vi "Get Physical Units from TD__ogtk.vi"(8 "error in (no error)":errorcluster, 10 "Float or Array Type Descriptor":T2) -> (0 "error out":errorcluster, 2 "Physical Units":T1[](array[typedef]))   [LabVIEW 2011]
doc: "Returns the physical units of the TD (number or array)."
uses:
  Type Descriptor__ogtk.ctl
  Physical Units__ogtk.ctl
panel:
  in  "Physical Units (type)":T1
  # "[OpenG VI Tags] ***Do Not Remove***"
  # "Please visit http://www.OpenG.org to learn about the\nOpen Source LabVIEW software movement.\n\nNOTICE -- YOU MUST LEAVE THIS NOTICE IN PLACE.  PER THE TERMS OF THE LICENSE BELOW, YOU MAY SUBLICENSE THIS SOFTWARE \nIN ANY WAY THAT DOES NOT CONFLICT WITH THIS LICENSE.\n\n### BSD License (http://www.opensource.org/licenses/bsd-license.php) Begin ###\n \nCopyright (c) 2002, Jean-Pierre Drolet <drolet_jp@hotmail.com>\nCopyright (c) 2002-2006, Jim Kring <jim@jimkring.com>\n\nAll rights reserved.\n\nRedistribution and use in source and binary forms, with or without modification, are permitted provided that the following conditions are met:\n\n    * Redistributions of source code must retain the above copyright notice, this list of conditions and the following disclaimer.\n    * Redistributions in binary form must reproduce the above copyright notice, this list of conditions and the following disclaimer in the \n       documentation and/or other materials provided with the distribution.\n    * Neither the name of SciWare, James Kring, Inc., nor the names of its contributors may be used to endorse or promote products derived \n       from this software without specific prior written permission.\n\nTHIS SOFTWARE IS PROVIDED BY THE COPYRIGHT HOLDERS AND CONTRIBUTORS \"AS IS\" AND ANY EXPRESS OR IMPLIED WARRANTIES, \nINCLUDING, BUT NOT LIMITED TO, THE IMPLIED WARRANTIES OF MERCHANTABILITY AND FITNESS FOR A PARTICULAR PURPOSE ARE \nDISCLAIMED. IN NO EVENT SHALL THE COPYRIGHT OWNER OR CONTRIBUTORS BE LIABLE FOR ANY DIRECT, INDIRECT, INCIDENTAL,\n SPECIAL, EXEMPLARY, OR CONSEQUENTIAL DAMAGES (INCLUDING, BUT NOT LIMITED TO, PROCUREMENT OF SUBSTITUTE GOODS OR \nSERVICES; LOSS OF USE, DATA, OR PROFITS; OR BUSINESS INTERRUPTION) HOWEVER CAUSED AND ON ANY THEORY OF LIABILITY, \nWHETHER IN CONTRACT, STRICT LIABILITY, OR TORT (INCLUDING NEGLIGENCE OR OTHERWISE) ARISING IN ANY WAY OUT OF THE USE \nOF THIS SOFTWARE, EVEN IF ADVISED OF THE POSSIBILITY OF SUCH DAMAGE.\n\n### BSD License End ###"
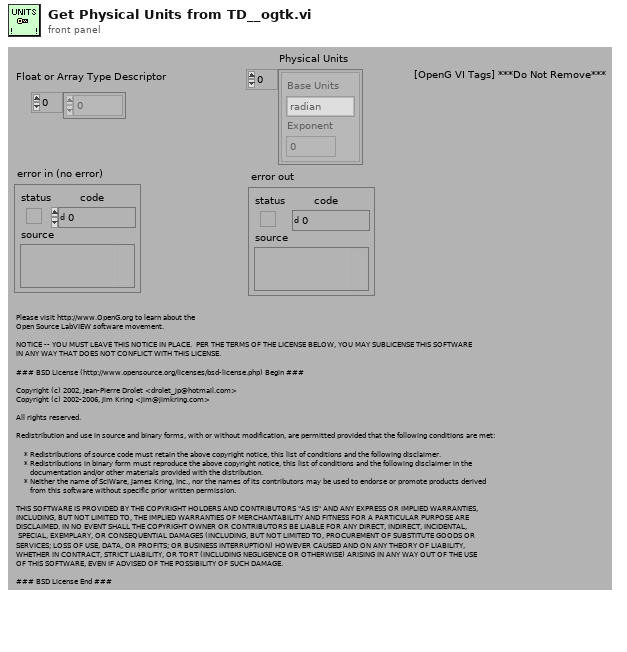
[diagram p1: front panel]
types:
  T1 = typedef "Physical Units__ogtk.ctl" = cluster{"Base Units":enum16{"radian", "steradian", "second", "meter", "kilogram", "ampere", "kelvin", "mole", "candela"}, "Exponent":i16}
  T2 = typedef "Type Descriptor__ogtk.ctl" = i16[]
  T3 = cluster{"Base Units":enum16{"radian", "steradian", "second", "meter", "kilogram", "ampere", "kelvin", "mole", "candela"}, "Exponent":i16}[]
  T4 = typedef "Type Descriptor Enumeration__ogtk.ctl" = enum8{"<Null>", "I8", "I16", "I32", "I64", "U8", "U16", "U32", "U64", "SGL", "DBL", "EXT", "CSG", "CDB", "CXT", "0x0F", "0x10", "0x11", "0x12", "0x13", "0x14", "Enum U8", "Enum U16", "Enum U32", "Enum U64", "SGL PQ", "DBL PQ", "EXT PQ", "CSG PQ", "CDB PQ", "CXT PQ", "0x1F", "0x20", "Boolean", "0x22", "0x23", "0x24", "0x25", "0x26", "0x27", "0x28", "0x29", "0x2A", "0x2B", "0x2C", "0x2D", "0x2E", "0x2F", "String", "0x31", "Path", "Pict", "0x34", "0x35", "0x36", "DAQ", "0x38", "0x39", "0x3A", "0x3B", "0x3C", "0x3D", "0x3E", "0x3F", "Array", "0x41", "0x42", "0x43", "0x44", "0x45", "0x46", "0x47", "0x48", "0x49", "0x4A", "0x4B", "0x4C", "0x4D", "0x4E", "0x4F", "Cluster", "0x51", "0x52", "Variant", "Waveform", "0x55", "0x56", "0x57", "0x58", "0x59", "0x5A", "0x5B", "0x5C", "0x5D", "0x5E", "0x5F", "0x60", "0x61", "0x62", "0x63", "0x64", "0x65", "0x66", "0x67", "0x68", "0x69", "0x6A", "0x6B", "0x6C", "0x6D", "0x6E", "0x6F", "Refnum"}
  T5 = typedef "Type Descriptor Header__ogtk.ctl" = cluster{"length":u16, "private":u8, "type":T4, "# elements":u16}
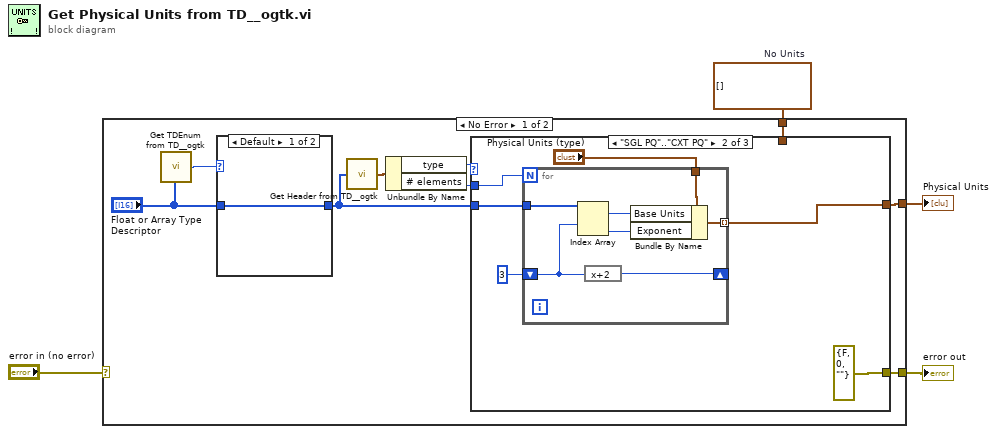
[diagram p0: block diagram]
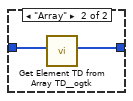
[diagram p2: hidden frame]
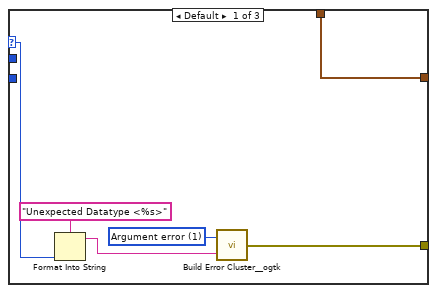
[diagram p3: hidden frame]
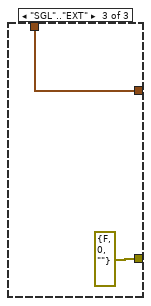
[diagram p4: hidden frame]
diagram:
  w1 = T3 []  # No Units
  n1 = case shown="No Error" "error in (no error)" {
    selector: "error in (no error)" -> [_ w39]
    tunnel: [w13 w39] -> w3
    tunnel: [w9 w38] -> w2
    tunnel: w1 -> [w8 w38]
    frame No Error {
      n2 = call "Get TDEnum from TD__ogtk.vi"("Type Descriptor"="Float or Array Type Descriptor") -> ("Type Descriptor Enumeration"=w7:T4)  [unwired: 4 in]
      n3 = case shown="Default" w7 {
        tunnel: "Float or Array Type Descriptor" -> [w14 w16]
        tunnel: [w14 w15] -> w5
        frame Default {
        }
        frame "Array" {
          n4 = call "Get Element TD from Array TD__ogtk.vi"("Array Type Descriptor"=w16) -> ("Element Type Descriptor"=w15:T2)  [unwired: 9 in, 1 out]
        }
      }
      n5 = call "Get Header from TD__ogtk.vi"("Type Descriptor"=w5) -> ("Type Descriptor Header"=w12:T5)
      n6 = Unbundle By Name(w12) -> ("type"=w11:T4, "# elements"=w10:u16)
      n7 = case shown="\"SGL PQ\"..\"CXT PQ\"" w11 {
        selector: w11 -> [w19 _ _]
        tunnel: [w22 errorcluster {"status"=FALSE, "code"=0, "source"=""} ("error out") errorcluster {"status"=FALSE, "code"=0, "source"=""} ("error out")] -> w13
        tunnel: w5 -> [_ w26 _]
        tunnel: w10 -> [_ w27 _]
        tunnel: [w17 w24 w37] -> w9
        tunnel: w8 -> [w17 _ w37]
        frame Default {
          w21 = 1 items=["No error", "Argument error", "Memory is full", "Out of zone", "End of file", "File already open", "Generic file I/O error", "File not found", "File permission error", "Disk is full", "Duplicate path", "Too many files open", "System feature not enabled", "Resource file not found", "Cannot add resource", "Resource not found", "Image not found", "Image memory error", "Pen does not exist", "Config type invalid", "Config token not found", "Config parse error", "Config memory error", "Bad external code format", "Bad external code offset", "External code not present", "Null window", "Destroy window error", "Null menu", "Print aborted", "Bad print record", "Print driver error", "Windows error during printing", "Memory error during printing", "Print dialog error", "Generic print error", "Invalid device refnum", "Device not found", "Device parameter error", "Device unit error", "Cannot open device", "Device call aborted", "Generic error", "Cancelled by user", "Object ID too low", "Object ID too high", "Object not in heap", "Unknown heap", "Unknown object (invalid DefProc)", "Unknown object (DefProc not in table)", "Message out of range", "Invalid (null) method", "Unknown message", "Manager call not supported", "Bad address", "Network operation in progress", "Network operation timed out", "Connection is busy", "Network attribute not supported", "Network error", "Address in use", "System out of memory", "Connection aborted", "Connection refused", "Not connected", "Already connected", "Connection closed", "Initialization error (interapplication manager)", "Bad occurrence", "Wait on unbound occurrence handler", "Occurrence queue overflow", "Datalog type conflict", "Unused", "Unrecognized type (interapplication manager)", "Memory corrupt", "Failed to make temporary DLL", "Old CIN version", "Drag socket not found", "Failed to load drop-object", "Failed to register OLE object", "Failed to release OLE object", "Format specifier type mismatch", "Unknown format specifier", "Too few format specifiers", "Too many format specifiers", "Scan failed", "Newer CIN version", "Error converting to variant", "Runtime menu error", "Password tampered", "Variant attribute not found", "Incompatible variant data type", "Event data is not available", "Event Store is not present", "Occurrence is not found", "Event Queue is not created", "Event info is not available", "Refnum passed is NULL", "Error retrieving Class GUID", "Error retrieving CoClass GUID", "Error retrieving TypeLib GUID.", "Bad built application magic bytes.", "Specific driver is different from the specific driver associated with the Logical Name.", "There is no session opened to the class driver.", "Max Error", "MAX - Error with config objects", "MAX - Error loading configuration", "MAX - Group not supported"]
          n8 = Format Into String(format string="Unexpected Datatype <%s>" ("Format String"), w19) -> (resulting string=w18:string)  [unwired: 2 in, 1 out]
          n9 = call "Build Error Cluster__ogtk.vi"("String to Prepend to source (\"\")"=w18, "code"=w21) -> ("error out"=w22:errorcluster)
        }
        frame "SGL PQ".."CXT PQ" {
          n10 = for {
            N: w27 -> [_]
            shift-right: [w30] -> _
            shift-left: 3 ("Index") -> [w31]
            tunnel: w26 -> [w35]
            tunnel: [w32] -> w24 mode=indexing
            tunnel: "Physical Units (type)" -> [w29]
            n11 = Index Array(array=w35, index #1=w31) -> (element #1=w33:i16, element #2=w34:i16)  [unwired: 1 in]
            n12 = expression code="x+2"(w31) -> (w30:i32)
            n13 = Bundle By Name(cluster=w29, "Base Units"=w33, "Exponent"=w34) -> (w32:T1)
          }
        }
        frame "SGL".."EXT" {
        }
      }
    }
    frame Error {
    }
  }
  "error out" <- w3
  "Physical Units" <- w2
